vi "host_get_lines.vi"(1 "in":string) -> (0 "out":string[](array[string]))   [LabVIEW 2021]
uses:
  <vilib>/regexp/Match Regular Expression.xnode
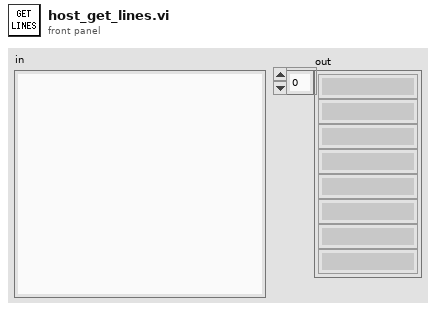
[diagram p1: front panel]
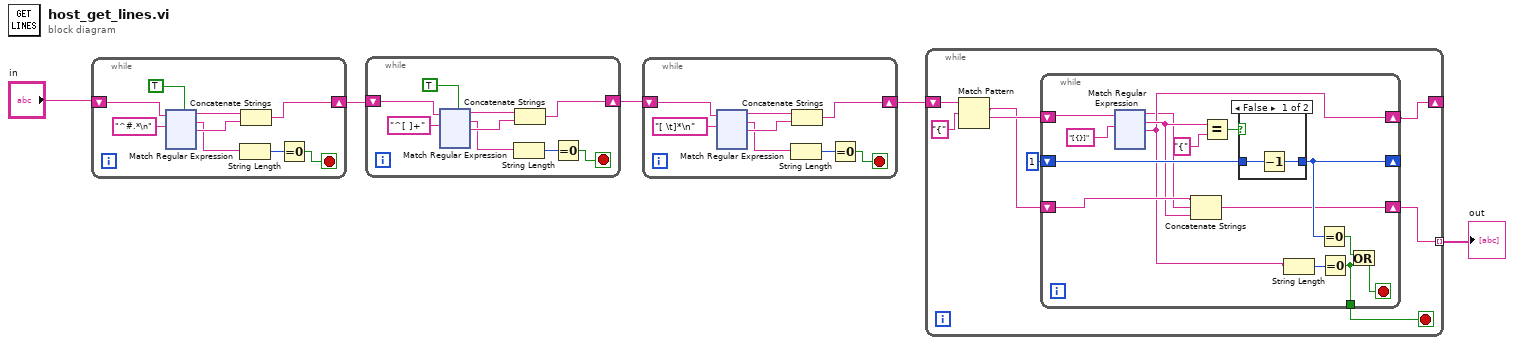
[diagram p0: block diagram]
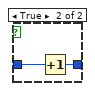
[diagram p2: hidden frame]
diagram:
  n1 = while {
    shift-right: [w7] -> w2
    shift-left: "in" -> [w13]
    stop <- w8 stop-if-true
    n2 = xnode "Match Regular Expression"("input string"=w13, "regular expression"="^#.*\n", "multiline? (F)"=TRUE) -> ("before match"=w12:string, "whole match"=w10:string, "after match"=w11:string)  [unwired: 3 in, 2 out]
    n3 = String Length(string=w10) -> (length=w9:i32)
    n4 = Concatenate Strings(w12, w11) -> (w7:string)
    n5 = Equal To 0?(x=w9) -> (x = 0?=w8:bool)
  }
  n6 = while {
    shift-right: [w133] -> w5
    shift-left: w2 -> [w139]
    stop <- w134 stop-if-true
    n7 = xnode "Match Regular Expression"("input string"=w139, "regular expression"="^[ ]+", "multiline? (F)"=TRUE) -> ("before match"=w138:string, "whole match"=w136:string, "after match"=w137:string)  [unwired: 3 in, 2 out]
    n8 = String Length(string=w136) -> (length=w135:i32)
    n9 = Concatenate Strings(w138, w137) -> (w133:string)
    n10 = Equal To 0?(x=w135) -> (x = 0?=w134:bool)
  }
  n11 = while {
    shift-right: [w258] -> w4
    shift-left: w5 -> [w264]
    stop <- w259 stop-if-true
    n12 = xnode "Match Regular Expression"("input string"=w264, "regular expression"="[ \t]*\n") -> ("before match"=w263:string, "whole match"=w261:string, "after match"=w262:string)  [unwired: 4 in, 2 out]
    n13 = String Length(string=w261) -> (length=w260:i32)
    n14 = Concatenate Strings(w263, w262) -> (w258:string)
    n15 = Equal To 0?(x=w260) -> (x = 0?=w259:bool)
  }
  n16 = while {
    tunnel: [w386] -> w3 mode=indexing
    shift-right: [w384] -> _
    shift-left: w4 -> [w385]
    stop <- w383 stop-if-true
    n17 = Match Pattern(string=w385, regular expression="{") -> (match substring=w387:string, after substring=w388:string)  [unwired: 1 in, 2 out]
    n18 = while {
      shift-right: [w398] -> _
      shift-left: 1 -> [w402]
      shift-right: [w394] -> w384
      shift-left: w388 -> [w391]
      shift-right: [w397] -> w386
      shift-left: w387 -> [w396]
      tunnel: [w393] -> w383
      stop <- w399 stop-if-true
      n19 = xnode "Match Regular Expression"("input string"=w391, "regular expression"="[{}]") -> ("before match"=w392:string, "whole match"=w395:string, "after match"=w394:string)  [unwired: 4 in, 2 out]
      n20 = Concatenate Strings(w396, w392, w395) -> (w397:string)
      n21 = Equal?(x=w395, y="{") -> (x = y?=w403:bool)
      n22 = case shown="False" w403 {
        tunnel: w402 -> [w524 w526]
        tunnel: [w523 w525] -> w398
        frame False {
          n23 = Decrement(x=w524) -> (x-1=w523:i32)
        }
        frame True {
          n24 = Increment(x=w526) -> (x+1=w525:i32)
        }
      }
      n25 = String Length(string=w394) -> (length=w400:i32)
      n26 = Equal To 0?(x=w398) -> (x = 0?=w401:bool)
      n27 = Equal To 0?(x=w400) -> (x = 0?=w393:bool)
      n28 = Or(x=w401, y=w393) -> (x .or. y?=w399:bool)
    }
  }
  "out" <- w3
